vi "Static Pattern.vi"(8 "error in (no error)":errorcluster, 10 "write data (0x0000)":u32, 11 "channel list (all:\"\")":string) -> (0 "error out":errorcluster)   [LabVIEW 2019]
uses:
  <instrlib>/niHSDIO/niHSDIO.llb/niHSDIO_ctl Voltage Logic Family Values (Ring).ctl
  Globals.vi
  <instrlib>/niHSDIO/niHSDIO.llb/niHSDIO Configure Data Voltage Logic Family.vi
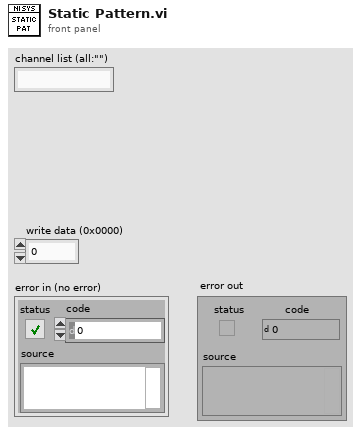
[diagram p1: front panel]
types:
  T1 = typedef "niHSDIO_ctl Voltage Logic Family Values (Ring).ctl" = i32
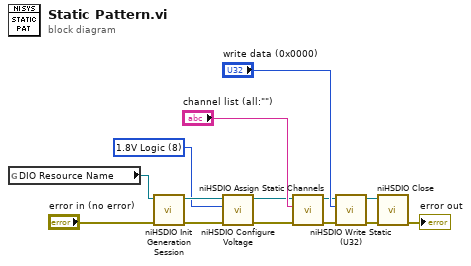
[diagram p0: block diagram]
diagram:
  w2 = T1 8 items=["5.0V Logic"=5, "3.3V Logic"=6, "2.5V Logic"=7, "1.8V Logic"=8, "1.5V Logic"=80, "1.2V Logic"=81] ("logic family (3.3V logic)")
  n1 = global read "Globals.vi" "DIO Resource Name"() -> (w1:refnum<k15>)
  n2 = call <instrlib>:"niHSDIO Init Generation Session.vi"("error in (no error)"="error in (no error)", "resource name"=w1) -> ("error out"=w4:errorcluster, "instrument handle out"=w6:refnum<k15>)  [unwired: 8 in]
  n3 = call-poly <instrlib>:"niHSDIO Configure Voltage.vi"("error in (no error)"=w4, "logic family (3.3V logic)"=w2, "instrument handle"=w6) -> ("error out"=w3:errorcluster, "instrument handle out"=w5:refnum<k15>)  [unwired: 7 in]
  n4 = call <instrlib>:"niHSDIO Assign Static Channels.vi"("error in (no error)"=w3, "channel list (all:\"\")"="channel list (all:\"\")", "instrument handle"=w5) -> ("error out"=w13:errorcluster, "instrument handle out"=w12:refnum<k15>)  [unwired: 7 in]
  n5 = call <instrlib>:"niHSDIO Write Static (U32).vi"("error in (no error)"=w13, "write data (0x0000)"="write data (0x0000)", "instrument handle"=w12) -> ("error out"=w9:errorcluster, "instrument handle out"=w7:refnum<k15>)  [unwired: 7 in]
  n6 = call <instrlib>:"niHSDIO Close.vi"("error in (no error)"=w9, "instrument handle"=w7) -> ("error out"=→"error out":errorcluster)  [unwired: 9 in]
